vi "Force Command Difference.vi"(0 "Target  Command Data In":T2, 1 "Previous  Measured Data In":T1, 2 "Current  Measured Data In":T1) -> (4 "Force Errors":dbl[](array[numeric]), 5 "Normalized Difference Vector":dbl[](array[numeric]), 6 "Force Commands Difference Vector":dbl[](array[numeric]))   [LabVIEW 2009]
uses:
  Target Data.ctl
  Data Access Objects/Metadata/LBCB Space.ctl
  Mixed Mode Cartesian Data.ctl
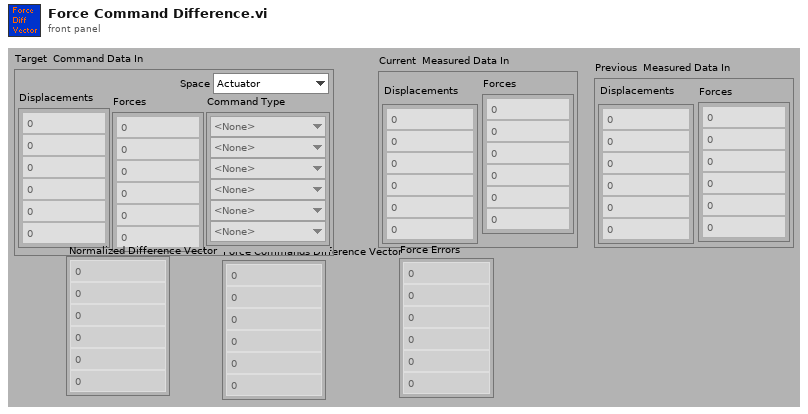
[diagram p1: front panel]
types:
  T1 = typedef "Mixed Mode Cartesian Data.ctl" = cluster{"Displacements":dbl[], "Forces":dbl[]}
  T2 = typedef "Target Data.ctl" = cluster{"Displacements":dbl[], "Command Type":enum16{"<None>", "Displacement", "Force"}[], "Forces":dbl[], "Space":T3}
  T3 = typedef "LBCB Space.ctl" = enum16{"Actuator", "Cartesian"}
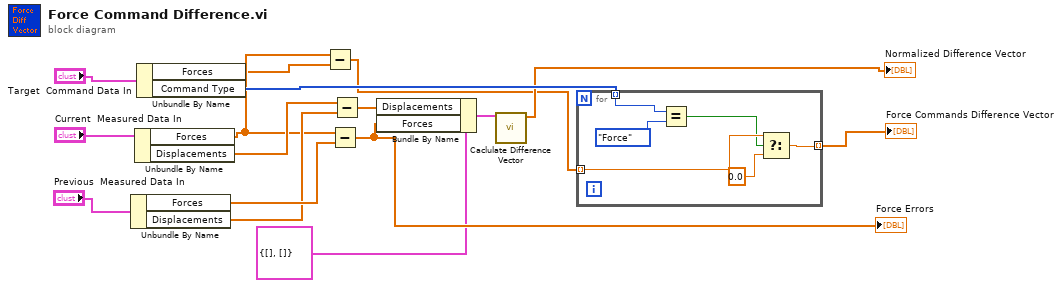
[diagram p0: block diagram]
diagram:
  n1 = Unbundle By Name("Previous  Measured Data In") -> ("Forces"=w6:dbl[], "Displacements"=w4:dbl[])
  n2 = Unbundle By Name("Current  Measured Data In") -> ("Forces"=w3:dbl[], "Displacements"=w5:dbl[])
  n3 = Unbundle By Name("Target  Command Data In") -> ("Forces"=w2:dbl[], "Command Type"=w11:enum16{"<None>", "Displacement", "Force"}[])
  n4 = Subtract(x=w3, y=w2) -> (x-y=w1:dbl[])
  n5 = Subtract(x=w3, y=w6) -> (x-y=w16:dbl[])
  "Force Errors" <- w16
  n6 = Subtract(x=w5, y=w4) -> (x-y=w15:dbl[])
  n7 = Bundle By Name(cluster=T1 {"Displacements"=[], "Forces"=[]} ("Increment In"), "Displacements"=w15, "Forces"=w16) -> (w14:T1)
  n8 = call "Caclulate Difference Vector.vi"("Increment In"=w14) -> ("Normalized Difference Vector"=→"Normalized Difference Vector":dbl[])  [unwired: 10 out]
  n9 = for {
    tunnel: w1 -> [w22] mode=indexing
    tunnel: w11 -> [w19] mode=indexing
    tunnel: [w20] -> w12 mode=indexing
    n10 = Equal?(x=w19, y=enum16{"<None>", "Displacement", "Force"}."Force") -> (x = y?=w18:bool)
    n11 = Select(t=w22, s=w18, f=0.0) -> (s? t:f=w20:dbl)
  }
  "Force Commands Difference Vector" <- w12
